vi "SeCrTs-RT_DAQ.vi"(8 "error in":errorcluster, 9 "er":refnum<queue>, 11 "Data FIFO Ref":T1) -> (0 "error out":errorcluster)   [LabVIEW 2022 SP3]
uses:
  RT Controls/SeCrTs-Data FIFO.ctl
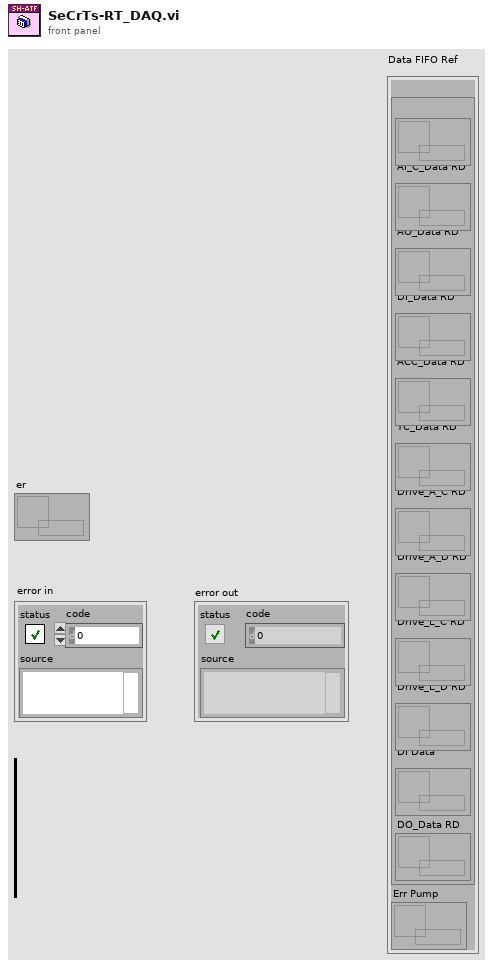
[diagram p1: front panel]
types:
  T1 = typedef "SeCrTs-Data FIFO.ctl" = cluster{"RD":cluster{"AI_V_Data RD":refnum<queue>, "AI_C_Data RD":refnum<queue>, "AO_Data RD":refnum<queue>, "DI_Data RD":refnum<queue>, "ACC_Data RD":refnum<queue>, "TC_Data RD":refnum<queue>, "Drive_A_C RD":refnum<queue>, "Drive_A_D RD":refnum<queue>, "Drive_L_C RD":refnum<queue>, "Drive_L_D RD":refnum<queue>, "DI Data":refnum<queue>, "DO_Data RD":refnum<queue>}, "Err Pump":refnum<queue>}
  T2 = cluster{"AO config":cluster{"Channel_Name":string, "Channel_Number":string, "Default_Value":dbl, "Units":string}[], "AI config":cluster{"Channel_Name":string, "Channel_Number":string, "Pre_Scale_min":dbl, "Pre_Scale_max":dbl, "Sensor_min":dbl, "Sensor_max":dbl, "Units":string}[], "DI config":cluster{"Channel_Name":string, "Channel_Number":string, "Default_Value":bool, "DI invert?":bool}[], "DO config":cluster{"Channel_Name":string, "Channel_Number":string, "Default_Value":bool, "DO invert?":bool}[], "TC config":cluster{"Channel_Name":string, "Channel_Number":string, "Pre_Scale_min":dbl, "Pre_Scale_max":dbl, "units":i32, " type":i32}[], "ACC config":cluster{"Channel_Name":string, "Channel_Number":string, "Pre_Scale_min":dbl, "Pre_Scale_max":dbl, "Terminal configuration":i32, "Sensitivity":dbl, "Sensitivity units":i32}[], "SG config":cluster{"Channel_Name":string, "Channel_Number":string, "Pre_Scale_min":dbl, "Pre_Scale_max":dbl}[], "Strain Gauge Settings":cluster{"poisson ratio":dbl, "nominal gage resistance":dbl, "gage factor":dbl}, "Bridge Settings":cluster{"voltage excitation value":dbl, "voltage excitation source":i32, "initial bridge voltage":dbl, "lead wire resistance":dbl, "strain configuration":i32}, "Sample Rate":cluster{"AI Sample Rate":dbl[], "AO Sample Rate":dbl[], "DI Sample Rate":dbl[], "TC Sample Rate":dbl[], "DO Sample Rate":dbl[], "SG Sample Rate":dbl[], "ACC Sample Rate":dbl[]}}
  T3 = enum16{"Initialize", "Create Task", "Start", "Acquire", "Stop", "Exit"}
  T4 = cluster{"AI_Task":refnum<k21>, "AO_Task":refnum<k21>, "DI_Task":refnum<k21>, "DO_Task":refnum<k21>, "ACC_Task":refnum<k21>, "TC_Task":refnum<k21>, "AI_V_Task":refnum<k21>}
  T5 = cluster{"Start DAQ":bool, "Stop DAQ":bool, "RT Stop":bool, "RT Exit":bool, "Start Seq":bool}
  T6 = cluster{"AO config":cluster{"Channel_Name":string, "Channel_Number":string, "Default_Value":dbl, "Units":string}[], "AI config":cluster{"Channel_Name":string, "Channel_Number":string, "Pre_Scale_min":dbl, "Pre_Scale_max":dbl, "Sensor_min":dbl, "Sensor_max":dbl, "Units":string}[], "DI config":cluster{"Channel_Name":string, "Channel_Number":string, "Default_Value":bool, "DI invert?":bool}[], "DO config":cluster{"Channel_Name":string, "Channel_Number":string, "Default_Value":bool, "DO invert?":bool}[], "TC config":cluster{"Channel_Name":string, "Channel_Number":string, "Pre_Scale_min":dbl, "Pre_Scale_max":dbl, "units":i32, "thermocouple type":i32}[], "ACC config":cluster{"Channel_Name":string, "Channel_Number":string, "Pre_Scale_min":dbl, "Pre_Scale_max":dbl, "Terminal configuration":i32, "Sensitivity":dbl, "Sensitivity units":i32}[], "SG config":cluster{"Channel_Name":string, "Channel_Number":string, "Pre_Scale_min":dbl, "Pre_Scale_max":dbl}[], "Strain Gauge Settings":cluster{"poisson ratio":dbl, "nominal gage resistance":dbl, "gage factor":dbl}, "Bridge Settings":cluster{"voltage excitation value":dbl, "voltage excitation source":i32, "initial bridge voltage":dbl, "lead wire resistance":dbl, "strain configuration":i32}, "Sample Rate":cluster{"AI Sample Rate":dbl[], "AO Sample Rate":dbl[], "DI Sample Rate":dbl[], "TC Sample Rate":dbl[], "DO Sample Rate":dbl[], "SG Sample Rate":dbl[], "ACC Sample Rate":dbl[]}}
  T7 = cluster{"Channel_Name":string, "Channel_Number":string, "Pre_Scale_min":dbl, "Pre_Scale_max":dbl, "Sensor_min":dbl, "Sensor_max":dbl, "Units":string}[]
  T8 = cluster{"Channel_Name":string, "Channel_Number":string, "Default_Value":dbl, "Units":string}[]
  T9 = cluster{"Channel_Name":string, "Channel_Number":string, "Default_Value":bool, "DI invert?":bool}[]
  T10 = cluster{"Channel_Name":string, "Channel_Number":string, "Default_Value":bool, "DO invert?":bool}[]
  T11 = cluster{"Channel_Name":string, "Channel_Number":string, "Pre_Scale_min":dbl, "Pre_Scale_max":dbl, "Terminal configuration":i32, "Sensitivity":dbl, "Sensitivity units":i32}[]
  T12 = cluster{"Channel_Name":string, "Channel_Number":string, "Pre_Scale_min":dbl, "Pre_Scale_max":dbl, "units":i32, " type":i32}[]
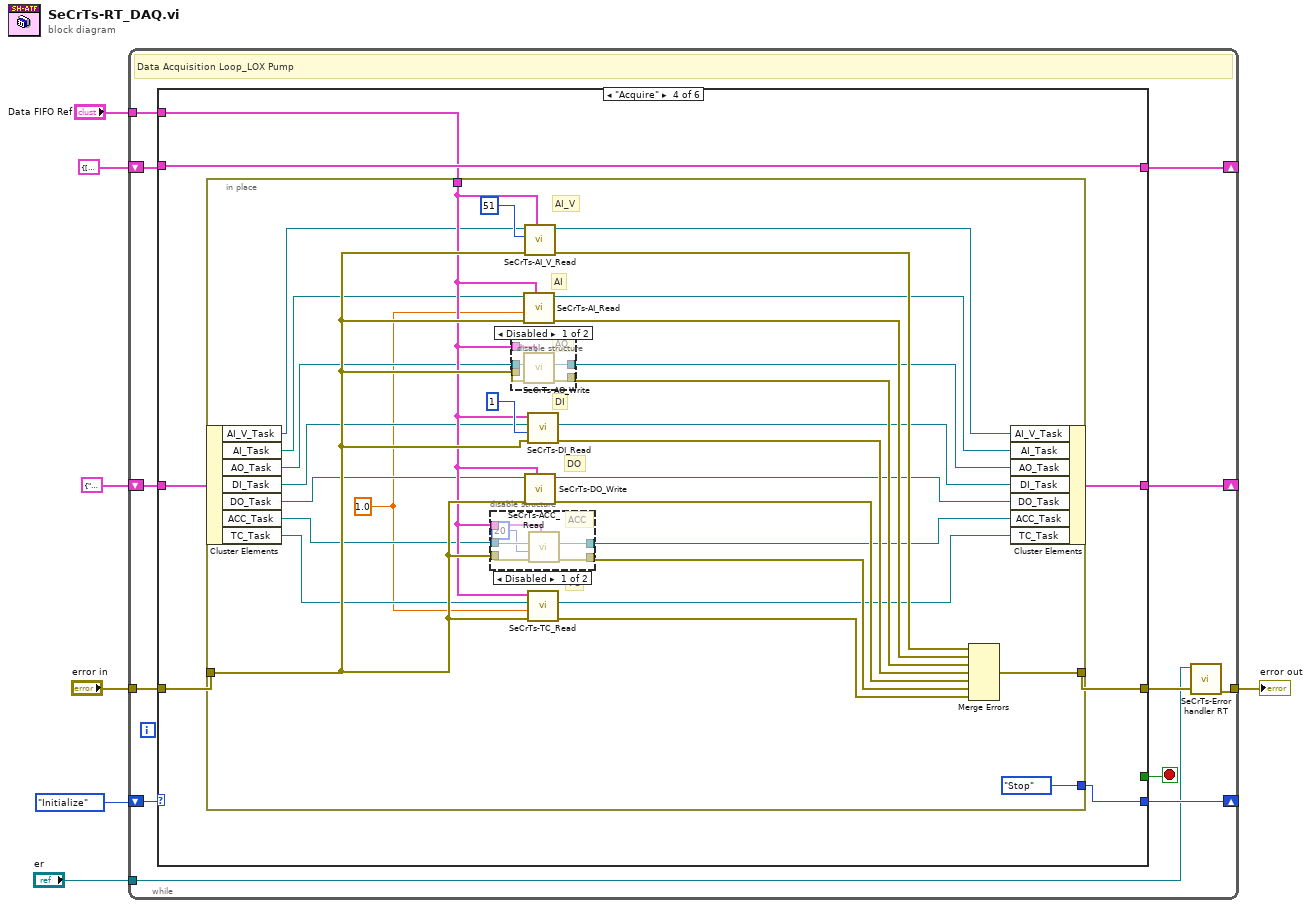
[diagram p0: block diagram]
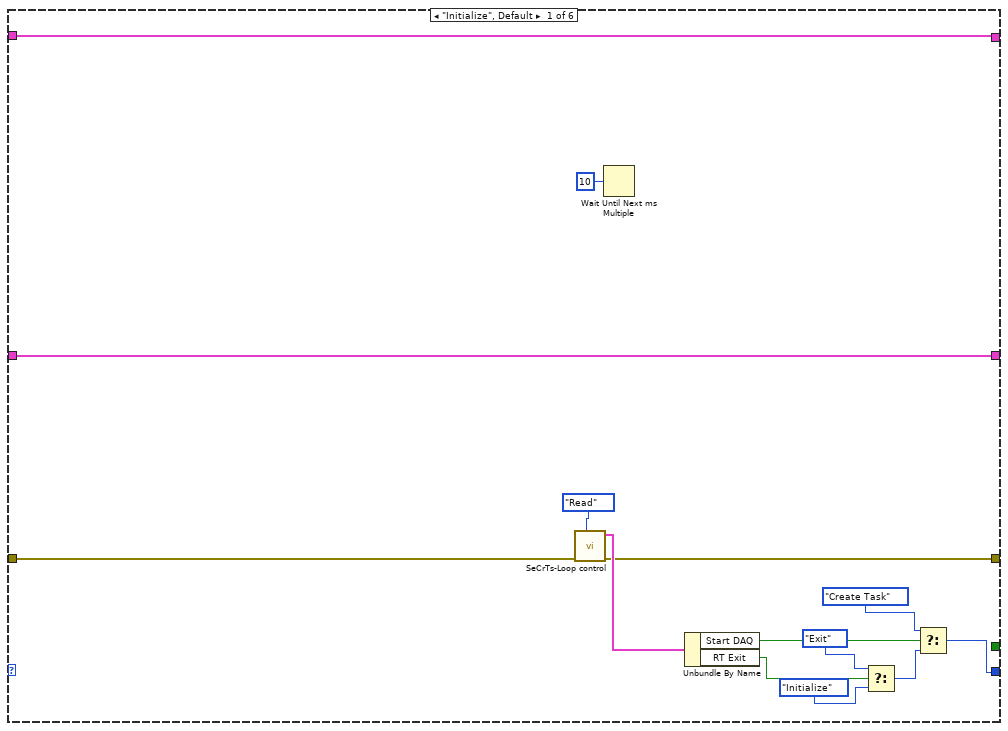
[diagram p2: hidden frame]
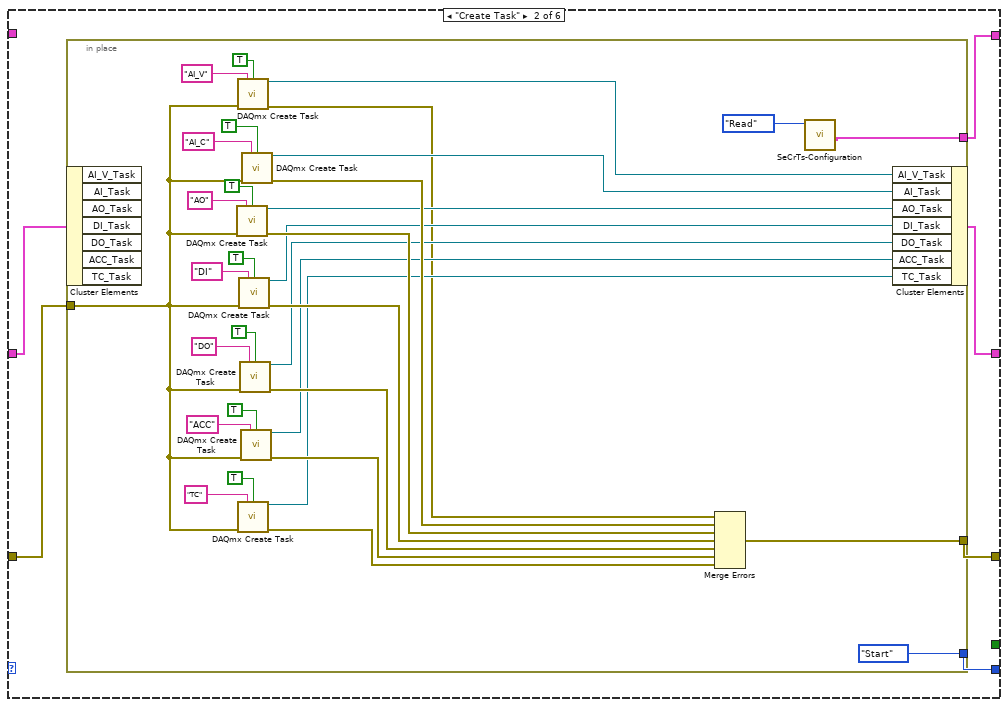
[diagram p3: hidden frame]
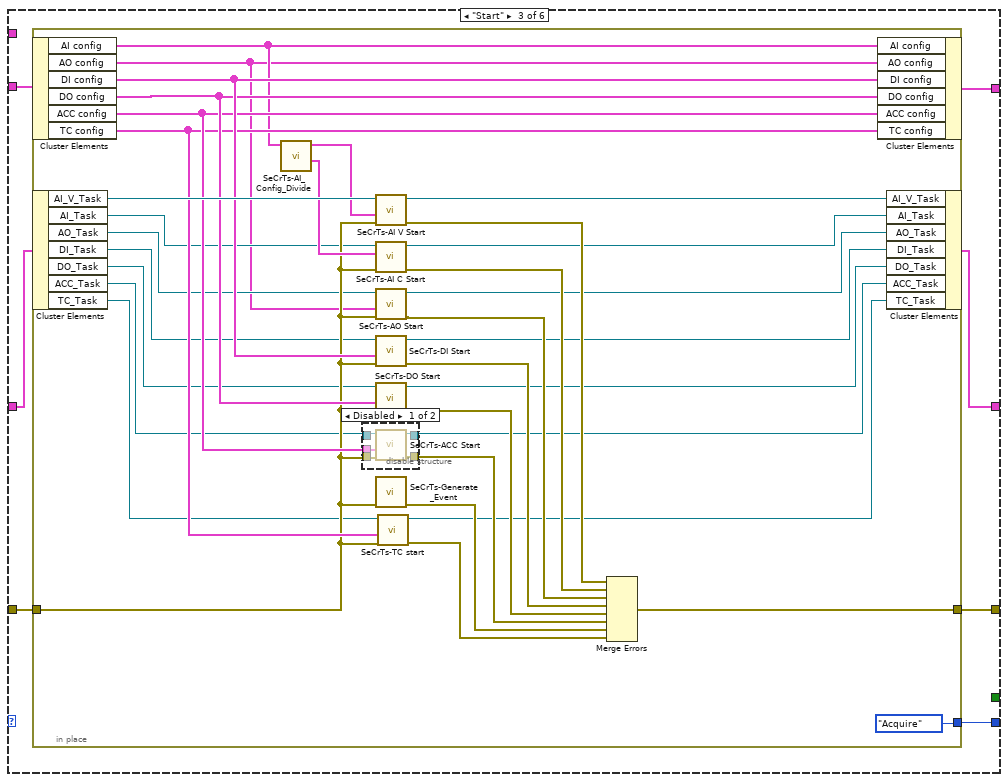
[diagram p4: hidden frame]
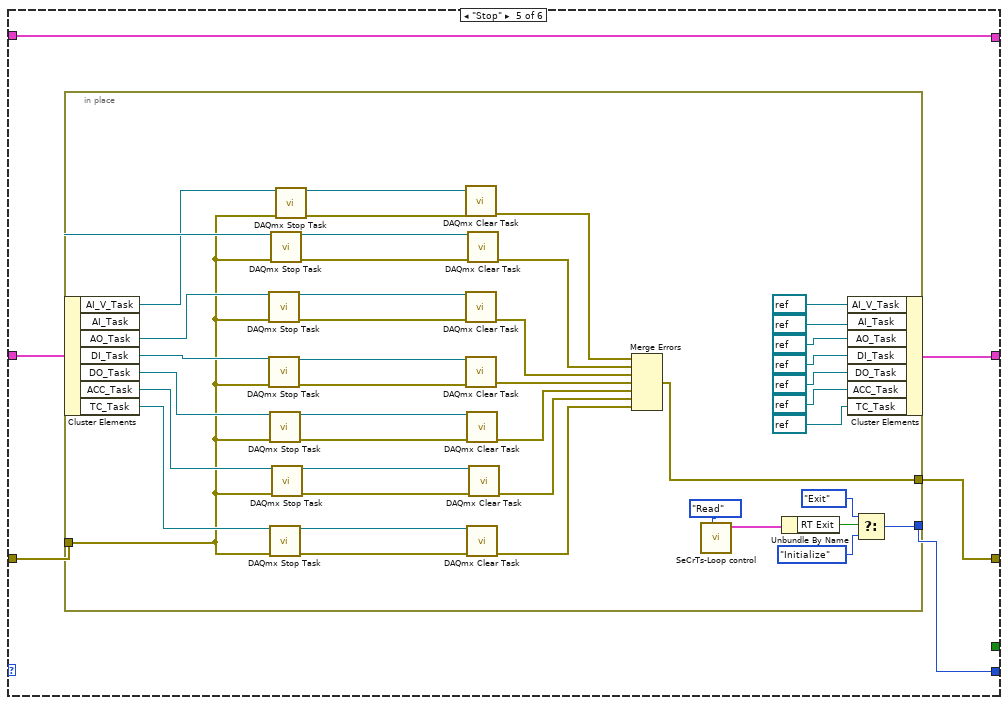
[diagram p8: hidden frame]
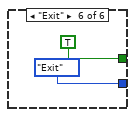
[diagram p9: hidden frame]
diagram:
  n1 = while {
    shift-right: [w17] -> _
    shift-left: T3."Initialize" -> [w19]
    tunnel: "error in" -> [w18]
    tunnel: [w8] -> w6
    shift-right: [w14] -> _
    shift-left: T2 {"AO config"=[], "AI config"=[], "DI config"=[], "DO config"=[], "TC config"=[], "ACC config"=[], "SG config"=[], "Strain Gauge Settings"={"poisson ratio"=0.0, "nominal gage resistance"=0.0, "gage factor"=0.0}, "Bridge Settings"={"voltage excitation value"=0.0, "voltage excitation source"=0, "initial bridge voltage"=0.0, "lead wire resistance"=0.0, "strain configuration"=0}, "Sample Rate"={"AI Sample Rate"=[], "AO Sample Rate"=[], "DI Sample Rate"=[], "TC Sample Rate"=[], "DO Sample Rate"=[], "SG Sample Rate"=[], "ACC Sample Rate"=[]}} ("Config out") -> [w15]
    shift-right: [w12] -> _
    shift-left: T4 {"AI_Task"="", "AO_Task"="", "DI_Task"="", "DO_Task"="", "ACC_Task"="", "TC_Task"="", "AI_V_Task"=""} -> [w16]
    tunnel: "Data FIFO Ref" -> [w11]
    tunnel: "er" -> [w9]
    stop <- w13 stop-if-true
    # "Data Acquisition Loop_LOX Pump"
    n2 = case shown="\"Acquire\"" w19 {
      tunnel: w18 -> [w22 w38 w78 w123 w167 _]
      tunnel: [w21 w37 w74 w122 w168 _] -> w10
      tunnel: [w32 w36 w79 w124 w169 T3."Exit"] -> w17
      tunnel: w16 -> [w24 w35 w77 w119 w166 _]
      tunnel: w15 -> [w23 _ w76 w121 w164 _]
      tunnel: [w23 w39 w75 w121 w164 _] -> w14
      tunnel: [_ _ _ _ _ TRUE] -> w13
      tunnel: [w24 w34 w73 w118 w165 _] -> w12
      tunnel: w11 -> [_ _ _ w120 _ _]
      frame "Initialize", Default {
        n3 = call "SeCrTs-Loop control.vi"("Action"=enum16{"Init", "Write", "Read"}."Read", "error in (no error)"=w22) -> ("error Out"=w21:errorcluster, "Loop Control out"=w28:T5)  [unwired: 8 in]
        n4 = Wait Until Next ms Multiple(millisecond multiple=u32 10) -> ()  [unwired: 1 out]
        n5 = Unbundle By Name(w28) -> ("Start DAQ"=w27:bool, "RT Exit"=w26:bool)
        n6 = Select(t=T3."Exit", s=w26, f=T3."Initialize") -> (s? t:f=w29:T3)
        n7 = Select(t=T3."Create Task", s=w27, f=w29) -> (s? t:f=w32:T3)
      }
      frame "Create Task" {
        n8 = in-place "In Place Element Structure" {
          in-place-border: [w51] -> w39
          in-place-border: w38 -> [w40]
          in-place-border: [w61] -> w37
          in-place-border: [T3."Start"] -> w36
          n9 = in-place-cluster #1(w35) -> ()  [unwired: 7 out]
          n10 = call <vilib>:"DAQmx Create Task.vi"("new task name"="AO", "auto cleanup"=TRUE, "error in"=w40) -> ("task out"=w59:refnum<k21>, "error out"=w66:errorcluster)  [unwired: 11 in]
          n11 = call <vilib>:"DAQmx Create Task.vi"("new task name"="AI_V", "auto cleanup"=TRUE, "error in"=w40) -> ("task out"=w52:refnum<k21>, "error out"=w41:errorcluster)  [unwired: 11 in]
          n12 = call <vilib>:"DAQmx Create Task.vi"("new task name"="TC", "auto cleanup"=TRUE, "error in"=w40) -> ("task out"=w55:refnum<k21>, "error out"=w62:errorcluster)  [unwired: 11 in]
          n13 = call <vilib>:"DAQmx Create Task.vi"("new task name"="DI", "auto cleanup"=TRUE, "error in"=w40) -> ("task out"=w58:refnum<k21>, "error out"=w65:errorcluster)  [unwired: 11 in]
          n14 = call <vilib>:"DAQmx Create Task.vi"("new task name"="DO", "auto cleanup"=TRUE, "error in"=w40) -> ("task out"=w57:refnum<k21>, "error out"=w64:errorcluster)  [unwired: 11 in]
          n15 = call <vilib>:"DAQmx Create Task.vi"("new task name"="ACC", "auto cleanup"=TRUE, "error in"=w40) -> ("task out"=w56:refnum<k21>, "error out"=w63:errorcluster)  [unwired: 11 in]
          n16 = call <vilib>:"DAQmx Create Task.vi"("new task name"="AI_C", "auto cleanup"=TRUE, "error in"=w40) -> ("task out"=w60:refnum<k21>, "error out"=w72:errorcluster)  [unwired: 11 in]
          n17 = Merge Errors(w41, w72, w66, w65, w64, w63, w62) -> (w61:errorcluster)
          n18 = call "SeCrTs-Configuration.vi"("Enum"=enum16{"Write", "Read"}."Read") -> ("Config out"=w51:T6)  [unwired: 10 in]
          n19 = in-place-cluster #1("AI_V_Task"=w52, "AI_Task"=w60, "AO_Task"=w59, "DI_Task"=w58, "DO_Task"=w57, "ACC_Task"=w56, "TC_Task"=w55) -> (w34:T4)
        }
      }
      frame "Start" {
        n20 = in-place "In Place Element Structure" {
          in-place-border: [T3."Acquire"] -> w79
          in-place-border: w78 -> [w98]
          in-place-border: [w93] -> w74
          n21 = in-place-cluster #2(w76) -> ("AI config"=w105:T7, "AO config"=w80:T8, "DI config"=w109:T9, "DO config"=w108:T10, "ACC config"=w107:T11, "TC config"=w106:T12)
          n22 = in-place-cluster #3(w77) -> ("AI_V_Task"=w111:refnum<k21>, "AI_Task"=w92:refnum<k21>, "AO_Task"=w91:refnum<k21>, "DI_Task"=w90:refnum<k21>, "DO_Task"=w89:refnum<k21>, "ACC_Task"=w88:refnum<k21>, "TC_Task"=w87:refnum<k21>)
          n23 = call "SeCrTs-AI_Config_Divide.vi"("AI config"=w105) -> ("AI C"=w103:T7, "AI V"=w104:T7)  [unwired: 9 in]
          n24 = disable-structure shown="Disabled" {
            disable-tunnel: w107 -> [w117 _]
            disable-tunnel: w98 -> [w116 _]
            disable-tunnel: [w115 _] -> w96
            disable-tunnel: w88 -> [w114 _]
            disable-tunnel: [w113 _] -> w82
            frame Disabled {
              n25 = call "SeCrTs-ACC Start.vi"("error in"=w116, "ACC config"=w117, "Refnum in"=w114) -> ("error out"=w115:errorcluster, "Refnum out"=w113:refnum<k21>)  [unwired: 7 in]
            }
            frame Enabled {
            }
          }
          n26 = call "SeCrTs-AI V Start .vi"("error in"=w98, "AI V"=w104, "Refnum in"=w111) -> ("error out"=w102:errorcluster, "Refnum out"=w110:refnum<k21>)  [unwired: 7 in]
          n27 = call "SeCrTs-AI C Start .vi"("error in"=w98, "AI C"=w103, "Refnum in"=w92) -> ("error out"=w101:errorcluster, "Refnum out"=w86:refnum<k21>)  [unwired: 7 in]
          n28 = call "SeCrTs-AO Start .vi"("error in"=w98, "AO config"=w80, "Refnum in"=w91) -> ("error out"=w100:errorcluster, "Refnum out"=w85:refnum<k21>)  [unwired: 7 in]
          n29 = call "SeCrTs-DI Start.vi"("error in"=w98, "DI config"=w109, "Refnum in"=w90) -> ("error out"=w99:errorcluster, "Refnum out"=w84:refnum<k21>)  [unwired: 7 in]
          n30 = call "SeCrTs-DO Start.vi"("error in"=w98, "DO config"=w108, "Refnum in"=w89) -> ("error out"=w97:errorcluster, "Refnum out"=w83:refnum<k21>)  [unwired: 7 in]
          n31 = call "SeCrTs-Generate_Event.vi"("error in"=w98) -> ("error out"=w95:errorcluster)  [unwired: 10 in]
          n32 = call "SeCrTs-TC start .vi"("error in"=w98, "TC config"=w106, "Refnum in"=w87) -> ("error out"=w94:errorcluster, "Refnum out"=w81:refnum<k21>)  [unwired: 7 in]
          n33 = Merge Errors(w102, w101, w100, w99, w97, w96, w95, w94) -> (w93:errorcluster)
          n34 = in-place-cluster #2("AI config"=w105, "AO config"=w80, "DI config"=w109, "DO config"=w108, "ACC config"=w107, "TC config"=w106) -> (w75:T2)
          n35 = in-place-cluster #3("AI_V_Task"=w110, "AI_Task"=w86, "AO_Task"=w85, "DI_Task"=w84, "DO_Task"=w83, "ACC_Task"=w82, "TC_Task"=w81) -> (w73:T4)
        }
      }
      frame "Acquire" {
        n36 = in-place "In Place Element Structure" {
          in-place-border: [T3."Stop"] -> w124
          in-place-border: w123 -> [w143]
          in-place-border: [w151] -> w122
          in-place-border: w120 -> [w141]
          w125 = 1.0
          # "AI_V"
          # "TC"
          # "DO"
          # "DI"
          # "AI"
          n37 = in-place-cluster #4(w119) -> ("AI_V_Task"=w126:refnum<k21>, "AI_Task"=w140:refnum<k21>, "AO_Task"=w139:refnum<k21>, "DI_Task"=w138:refnum<k21>, "DO_Task"=w137:refnum<k21>, "ACC_Task"=w136:refnum<k21>, "TC_Task"=w135:refnum<k21>)
          n38 = disable-structure shown="Disabled" {
            disable-tunnel: [w158 _] -> w145
            disable-tunnel: w143 -> [w157 _]
            disable-tunnel: w141 -> [w156 _]
            disable-tunnel: w136 -> [w155 _]
            disable-tunnel: [w154 _] -> w129
            frame Disabled {
              # "ACC"
              n39 = call "SeCrTs-ACC_Read.vi"("Data FIFO Ref"=w156, "error in (no error)"=w157, "number of samples per channel"=20, "ACC_Task"=w155) -> ("error out"=w158:errorcluster, "task out"=w154:refnum<k21>)  [unwired: 6 in]
            }
            frame Enabled {
            }
          }
          n40 = disable-structure shown="Disabled" {
            disable-tunnel: [w163 _] -> w148
            disable-tunnel: w143 -> [w162 _]
            disable-tunnel: w141 -> [w161 _]
            disable-tunnel: w139 -> [w160 _]
            disable-tunnel: [w159 _] -> w132
            frame Disabled {
              # "AO"
              n41 = call "SeCrTs-AO_Write.vi"("Data FIFO Ref"=w161, "error in (no error)"=w162, "AO_Task"=w160) -> ("error out"=w163:errorcluster, "task out"=w159:refnum<k21>)  [unwired: 7 in]
            }
            frame Enabled {
            }
          }
          n42 = call "SeCrTs-AI_Read.vi"("Data FIFO Ref"=w141, "error in (no error)"=w143, "Numeric"=w125, "AI_Task"=w140) -> ("error out"=w149:errorcluster, "task out"=w133:refnum<k21>)  [unwired: 4 in]
          n43 = call "SeCrTs-AI_V_Read.vi"("Data FIFO Ref"=w141, "error in"=w143, "number of samples per channel"=51, "AI_V_Task"=w126) -> ("error out"=w150:errorcluster, "AI_V_Task"=w134:refnum<k21>)  [unwired: 6 in]
          n44 = call "SeCrTs-DO_Write.vi"("Data FIFO Ref"=w141, "error in (no error)"=w143, "Refnum in"=w137) -> ("error out"=w146:errorcluster, "Refnum out"=w130:refnum<k21>)  [unwired: 7 in]
          n45 = call "SeCrTs-DI_Read.vi"("error in (no error)"=w143, "number of samples per channel"=1, "DI_Task"=w138, "Data FIFO Ref"=w141) -> ("error out"=w147:errorcluster, "task out"=w131:refnum<k21>)  [unwired: 6 in]
          n46 = call "SeCrTs-TC_Read.vi"("error in (no error)"=w143, "Numeric"=w125, "TC_Task"=w135, "Data FIFO Ref"=w141) -> ("error out"=w144:errorcluster, "task out"=w128:refnum<k21>)  [unwired: 6 in]
          n47 = Merge Errors(w150, w149, w148, w147, w146, w145, w144) -> (w151:errorcluster)
          n48 = in-place-cluster #4("AI_V_Task"=w134, "AI_Task"=w133, "AO_Task"=w132, "DI_Task"=w131, "DO_Task"=w130, "ACC_Task"=w129, "TC_Task"=w128) -> (w118:T4)
        }
      }
      frame "Stop" {
        n49 = in-place "In Place Element Structure" {
          in-place-border: [w209] -> w169
          in-place-border: [w203] -> w168
          in-place-border: w167 -> [w184]
          n50 = in-place-cluster #5(w166) -> ("AI_V_Task"=w186:refnum<k21>, "AI_Task"=w195:refnum<k21>, "AO_Task"=w194:refnum<k21>, "DI_Task"=w197:refnum<k21>, "DO_Task"=w196:refnum<k21>, "ACC_Task"=w193:refnum<k21>, "TC_Task"=w192:refnum<k21>)
          n51 = call <vilib>:"DAQmx Stop Task.vi"("task/channels in"=w194, "error in"=w184) -> ("task out"=w191:refnum<k21>, "error out"=w208:errorcluster)  [unwired: 12 in]
          n52 = call <vilib>:"DAQmx Stop Task.vi"("task/channels in"=w197, "error in"=w184) -> ("task out"=w190:refnum<k21>, "error out"=w207:errorcluster)  [unwired: 12 in]
          n53 = call <vilib>:"DAQmx Stop Task.vi"("task/channels in"=w196, "error in"=w184) -> ("task out"=w189:refnum<k21>, "error out"=w206:errorcluster)  [unwired: 12 in]
          n54 = call <vilib>:"DAQmx Stop Task.vi"("task/channels in"=w192, "error in"=w184) -> ("task out"=w187:refnum<k21>, "error out"=w204:errorcluster)  [unwired: 12 in]
          n55 = call <vilib>:"DAQmx Stop Task.vi"("task/channels in"=w195, "error in"=w184) -> ("task out"=w172:refnum<k21>, "error out"=w171:errorcluster)  [unwired: 12 in]
          n56 = call <vilib>:"DAQmx Stop Task.vi"("task/channels in"=w193, "error in"=w184) -> ("task out"=w188:refnum<k21>, "error out"=w205:errorcluster)  [unwired: 12 in]
          n57 = call <vilib>:"DAQmx Stop Task.vi"("task/channels in"=w186, "error in"=w184) -> ("task out"=w185:refnum<k21>, "error out"=w183:errorcluster)  [unwired: 12 in]
          n58 = call <vilib>:"DAQmx Clear Task.vi"("task in"=w185, "error in"=w183) -> ("error out"=w182:errorcluster)  [unwired: 13 in]
          n59 = call <vilib>:"DAQmx Clear Task.vi"("task in"=w191, "error in"=w208) -> ("error out"=w202:errorcluster)  [unwired: 13 in]
          n60 = call <vilib>:"DAQmx Clear Task.vi"("task in"=w190, "error in"=w207) -> ("error out"=w201:errorcluster)  [unwired: 13 in]
          n61 = call <vilib>:"DAQmx Clear Task.vi"("task in"=w189, "error in"=w206) -> ("error out"=w200:errorcluster)  [unwired: 13 in]
          n62 = call <vilib>:"DAQmx Clear Task.vi"("task in"=w187, "error in"=w204) -> ("error out"=w198:errorcluster)  [unwired: 13 in]
          n63 = call <vilib>:"DAQmx Clear Task.vi"("task in"=w172, "error in"=w171) -> ("error out"=w212:errorcluster)  [unwired: 13 in]
          n64 = call <vilib>:"DAQmx Clear Task.vi"("task in"=w188, "error in"=w205) -> ("error out"=w199:errorcluster)  [unwired: 13 in]
          n65 = Merge Errors(w182, w212, w202, w201, w200, w199, w198) -> (w203:errorcluster)
          n66 = call "SeCrTs-Loop control.vi"("Action"=enum16{"Init", "Write", "Read"}."Read") -> ("Loop Control out"=w181:T5)  [unwired: 9 in, 1 out]
          n67 = Unbundle By Name(w181) -> ("RT Exit"=w180:bool)
          n68 = in-place-cluster #5("AI_V_Task"=refnum<k21> refnum, "AI_Task"=refnum<k21> refnum, "AO_Task"=refnum<k21> refnum, "DI_Task"=refnum<k21> refnum, "DO_Task"=refnum<k21> refnum, "ACC_Task"=refnum<k21> refnum, "TC_Task"=refnum<k21> refnum) -> (w165:T4)
          n69 = Select(t=T3."Exit", s=w180, f=T3."Initialize") -> (s? t:f=w209:T3)
        }
      }
      frame "Exit" {
      }
    }
    n70 = call "SeCrTs-Error handler RT.vi"("error in"=w10, "Message Queue"=w9) -> ("error out"=w8:errorcluster)  [unwired: 8 in, 1 out]
  }
  "error out" <- w6
